vi "AR-GC-Stop-FGV.vi"(7 "Action (RD)":enum16{"Init", "WR", "RD"}(ring)=enum."RD", 10 "error in":errorcluster, 11 "Action":bool) -> (2 "error out":errorcluster, 3 "Out":bool)   [LabVIEW 2021]
doc: "Functional Global\n\nAvoids racing conditions. Used to convey Stop a loop message between multiple parallel loops.\n\nActions: Init, RD, WR"
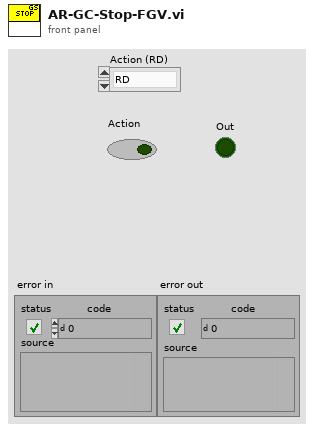
[diagram p1: front panel]
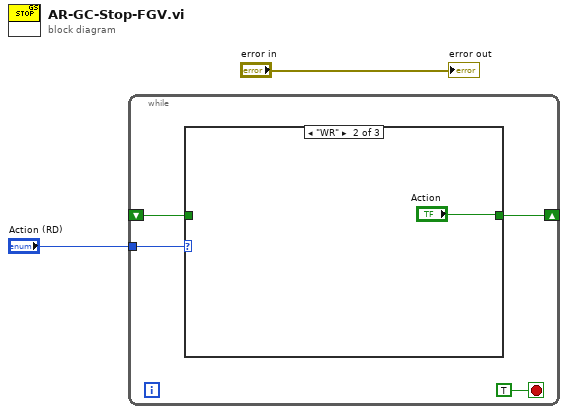
[diagram p0: block diagram]
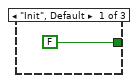
[diagram p2: hidden frame]
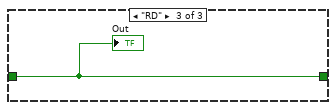
[diagram p3: hidden frame]
diagram:
  n1 = while {
    tunnel: "Action (RD)" -> [w6]
    shift-right: [w4] -> _
    shift-left: _ -> [w3]
    stop <- TRUE stop-if-true
    n2 = case shown="\"WR\"" w6 {
      tunnel: [FALSE ("Out") "Action" w9] -> w4
      tunnel: w3 -> [_ _ w9]
      frame "Init", Default {
      }
      frame "WR" {
      }
      frame "RD" {
        "Out" <- w9
      }
    }
  }
  "error out" <- "error in"
